vi "GetCRC8.vi"(8 "错误输入（无错误）":errorcluster, 11 "xData":u8[](array[numeric]) format="0x%x") -> (0 "错误输出":errorcluster, 3 "CRC8":u8 format="0x%x")   [LabVIEW 2020]
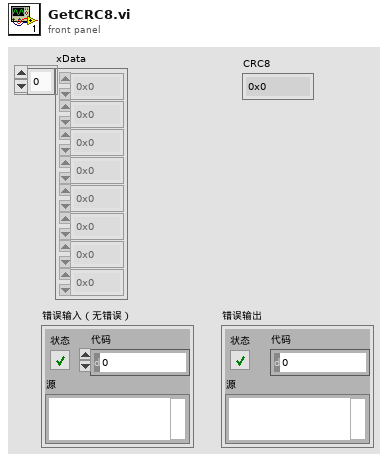
[diagram p1: front panel]
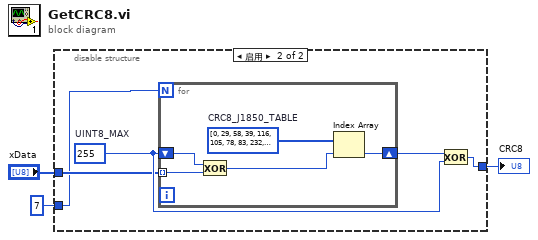
[diagram p0: block diagram]
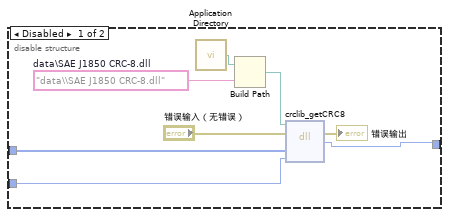
[diagram p2: hidden frame]
diagram:
  n1 = disable-structure shown="启用" {
    disable-tunnel: "xData" -> [w9 w14]
    disable-tunnel: u16 7 ("xDataLen") -> [w8 w13]
    disable-tunnel: [w7 w12] -> w1
    frame Disabled {
      w5 = "data\\SAE J1850 CRC-8.dll"  # data\SAE J1850 CRC-8.dll
      n2 = call <vilib>:"Application Directory.vi"() -> ("Application Directory"=w6:path)
      n3 = Build Path(base path=w6, name or relative path=w5) -> (appended path=w4:path)
      n4 = dll-call lib="PTH2Xabs CUsersFeng项目HLCEPS300-1老性能试验台dataSAE J1850 CRC-8.dll" fn="crclib_getCRC8"(path in=w4, error in="错误输入（无错误）", "xData"=w9, "xDataLen"=w8) -> (error out=→"错误输出":errorcluster, "返回类型"=w7:u8)  [unwired: 3 in, 1 out]
    }
    frame Enabled {
      w15 = u8 255  # UINT8_MAX
      n5 = for {
        N: w13 -> [_]
        shift-right: [w20] -> w16
        shift-left: w15 -> [w19]
        tunnel: w14 -> [w18] mode=indexing
        w21 = u8[] [0, 29, 58, 39, 116, 105, 78, 83, 232, 245, 210, 207, 156, 129, 166, 187, 205, 208, 247, 234, 185, 164, 131, 158, 37, 56, 31, 2, 81, 76, 107, 118, 135, 154, 189, 160, 243, 238, 201, 212, 111, 114, 85, 72, 27, 6, 33, 60, 74, 87, 112, 109, 62, 35, 4, 25, 162, 191, 152, 133, 214, 203, 236, 241, 19, 14, 41, 52, 103, 122, 93, 64, 251, 230, 193, 220, 143, 146, 181, 168, 222, 195, 228, 249, 170, 183, 144, 141, 54, 43, 12, 17, 66, 95, 120, 101, 148, 137, 174, 179, 224, 253, 218, 199, 124, 97, 70, 91, 8, 21, 50, 47, 89, 68, 99, 126, 45, 48, 23, 10, 177, 172, 139, 150, 197, 216, 255, 226, 38, 59, 28, 1, 82, 79, 104, 117, 206, 211, 244, 233, 186, 167, 128, 157, 235, 246, 209, 204, 159, 130, 165, 184, 3, 30, 57, 36, 119, 106, 77, 80, 161, 188, 155, 134, 213, 200, 239, 242, 73, 84, 115, 110, 61, 32, 7, 26, 108, 113, 86, 75, 24, 5, 34, 63, 132, 153, 190, 163, 240, 237, 202, 215, 53, 40, 15, 18, 65, 92, 123, 102, 221, 192, 231, 250, 169, 180, 147, 142, 248, 229, 194, 223, 140, 145, 182, 171, 16, 13, 42, 55, 100, 121, 94, 67, 178, 175, 136, 149, 198, 219, 252, 225, 90, 71, 96, 125, 46, 51, 20, 9, 127, 98, 69, 88, 11, 22, 49, 44, 151, 138, 173, 176, 227, 254, 217, 196]  # CRC8_J1850_TABLE
        n6 = Exclusive Or(1:w18, 2:w19) -> (0:w17:u8)
        n7 = Index Array(array=w21, index=w17) -> (element=w20:u8)
      }
      n8 = Exclusive Or(1:w15, 2:w16) -> (0:w12:u8)
    }
  }
  "CRC8" <- w1
